vi "AI and AO.vi"(8 "error in (no error)":errorcluster, 10 "AO":waveform(dbl)[](array[waveform]), 11 "LockinDAQ in":refnum<class "LockinDAQ.lvclass">) -> (0 "error out":errorcluster, 2 "AI":waveform(dbl)[](array[waveform]), 3 "LockinDAQ out":refnum<class "LockinDAQ.lvclass">)   [LabVIEW 2016, in "LockinDAQ.lvclass"]
uses:
  LockinDAQ.lvclass
  LockinDAQ.lvclass/LockinDAQ.ctl
  <vilib>/DAQmx/read.llb/DAQmx Read (Analog 1D Wfm NChan NSamp).vi
  <vilib>/DAQmx/write.llb/DAQmx Write (Analog 1D Wfm NChan NSamp).vi
  <vilib>/DAQmx/miscellaneous.llb/DAQmx Fill In Error Info.vi
  <resource>/objmgr/daqmx.rc
panel:
  out "AvailSampPerChan 4":u32
  out "AvailSampPerChan 3":u32
  out "AvailSampPerChan 2":u32
  out "AvailSampPerChan 1":u32
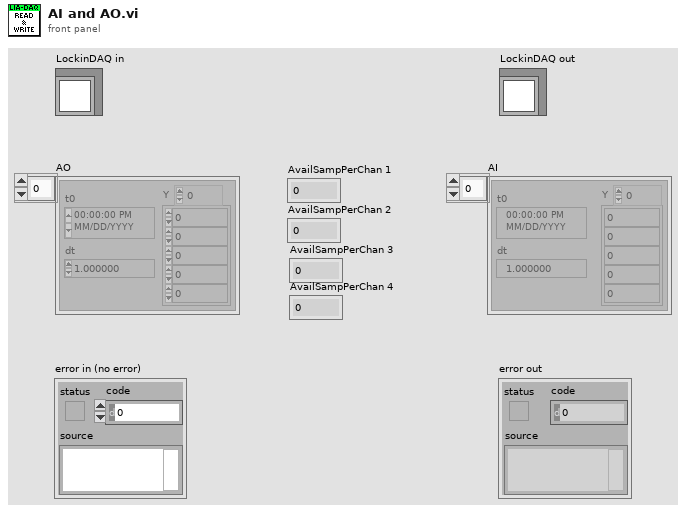
[diagram p1: front panel]
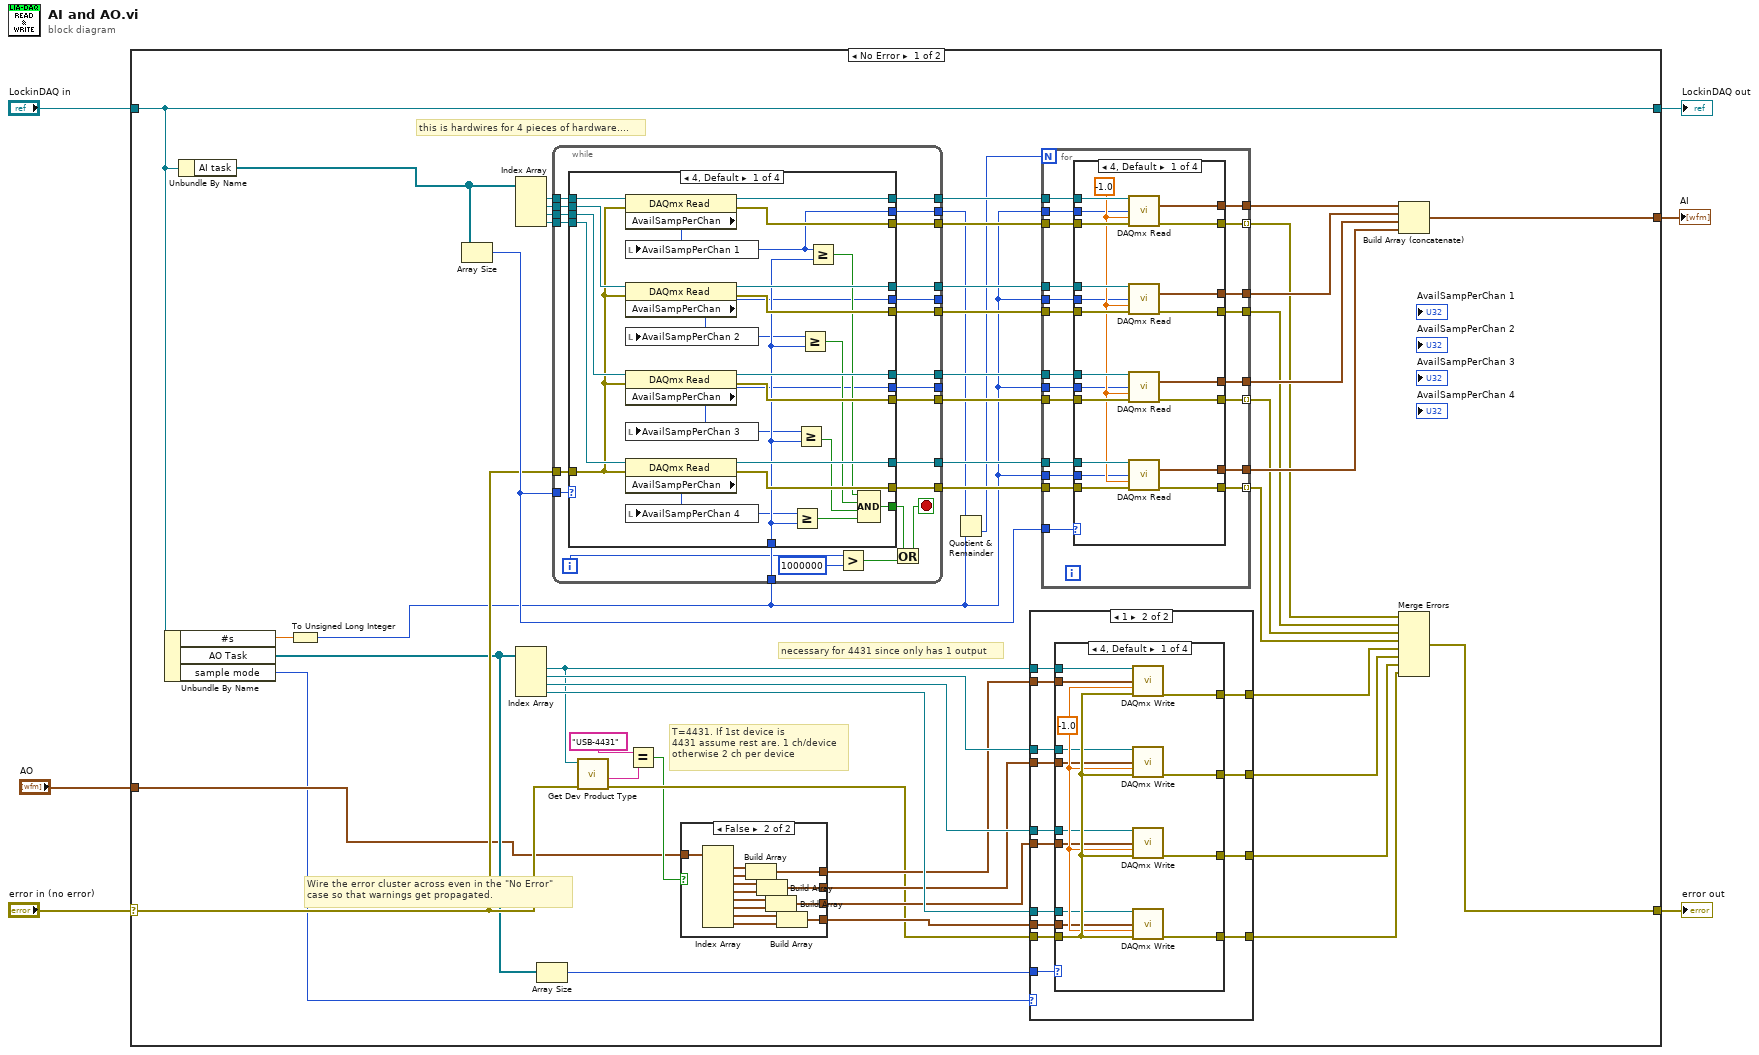
[diagram p0: block diagram]
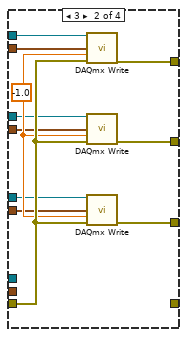
[diagram p3: hidden frame]
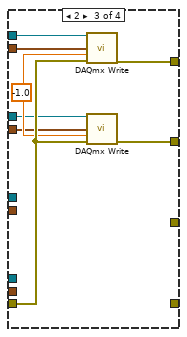
[diagram p4: hidden frame]
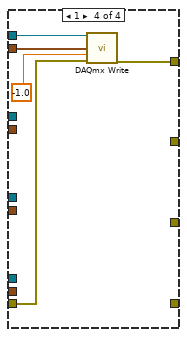
[diagram p5: hidden frame]
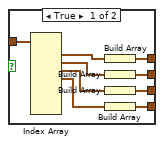
[diagram p6: hidden frame]
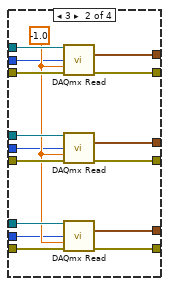
[diagram p7: hidden frame]
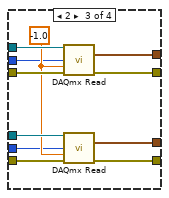
[diagram p8: hidden frame]
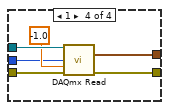
[diagram p9: hidden frame]
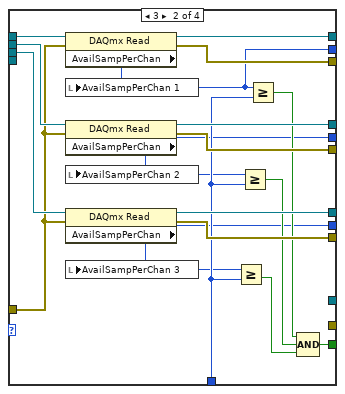
[diagram p10: hidden frame]
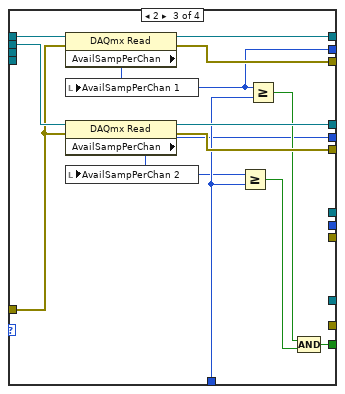
[diagram p11: hidden frame]
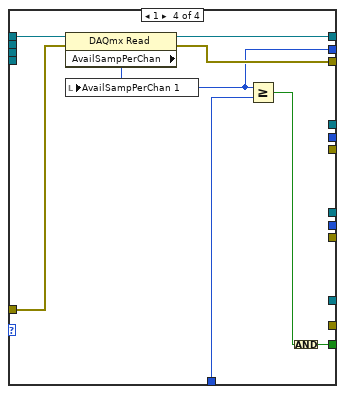
[diagram p12: hidden frame]
diagram:
  n1 = case shown="No Error" "error in (no error)" {
    selector: "error in (no error)" -> [w16 w292]
    tunnel: [w15 w292] -> w5
    tunnel: [w13 w291] -> w3
    tunnel: "LockinDAQ in" -> [w13 w291]
    tunnel: "AO" -> [w11 _]
    tunnel: [w10 _] -> w1
    frame No Error {
      # "this is hardwires for 4 pieces of hardware...."
      # "T=4431. If 1st device is \n4431 assume rest are. 1 ch/device\notherwise 2 ch per device"
      # "necessary for 4431 since only has 1 output"
      # "Wire the error cluster across even in the \"No Error\"\ncase so that warnings get propagated."
      n2 = Unbundle By Name(w13) -> ("#s"=w9:dbl, "AO Task"=w12:refnum<k21>[], "sample mode"=w7:i32)
      n3 = Unbundle By Name(w13) -> ("AI task"=w14:refnum<k21>[])
      n4 = To Unsigned Long Integer(number=w9) -> (unsigned 32bit integer=w8:u32)
      n5 = Array Size(array=w14) -> (size(s)=w21:i32)
      n6 = Index Array(array=w14) -> (element #1=w53:refnum<k21>, element #2=w54:refnum<k21>, element #3=w55:refnum<k21>, element #4=w56:refnum<k21>)  [unwired: 4 in]
      n7 = Index Array(array=w12) -> (element #1=w30:refnum<k21>, element #2=w44:refnum<k21>, element #3=w43:refnum<k21>, element #4=w42:refnum<k21>)  [unwired: 4 in]
      n8 = Array Size(array=w12) -> (size(s)=w31:i32)
      n9 = while {
        tunnel: w56 -> [w228]
        tunnel: w55 -> [w227]
        tunnel: w54 -> [w226]
        tunnel: w53 -> [w225]
        tunnel: [w224] -> w52
        tunnel: [w223] -> w51
        tunnel: [w222] -> w50
        tunnel: [w221] -> w49
        tunnel: w16 -> [w216]
        tunnel: [w220] -> w48
        tunnel: [w219] -> w47
        tunnel: [w218] -> w46
        tunnel: [w217] -> w45
        tunnel: w8 -> [w215]
        tunnel: [w212] -> w32
        tunnel: [w214] -> _
        tunnel: [w213] -> _
        tunnel: w21 -> [w211]
        i -> [w208]
        stop <- w209 stop-if-true
        n10 = case shown="4, Default" w211 {
          tunnel: w228 -> [w251 _ _ _]
          tunnel: w227 -> [w250 w269 _ _]
          tunnel: w226 -> [w249 w268 w282 _]
          tunnel: w225 -> [w248 w267 w281 w290]
          tunnel: [w247 w266 w280 w289] -> w224
          tunnel: [w246 w265 w279 _] -> w223
          tunnel: [w245 w264 _ _] -> w222
          tunnel: [w244 _ _ _] -> w221
          tunnel: [w243 w263 w278 w288] -> w220
          tunnel: [w242 w262 w277 _] -> w219
          tunnel: [w241 w261 _ _] -> w218
          tunnel: [w240 _ _ _] -> w217
          tunnel: w216 -> [w239 w260 w276 w287]
          tunnel: w215 -> [w234 w256 w273 w285]
          tunnel: [w229 w252 w270 w283] -> w210
          tunnel: [w232 w255 _ _] -> w214
          tunnel: [w231 w254 w272 _] -> w213
          tunnel: [w230 w253 w271 w284] -> w212
          frame 4, Default {
            n11 = property class="DAQmx Read"(reference=w248, error in=w239) -> (reference out=w247:refnum<k21>, error out=w243:errorcluster, "AvailSampPerChan"=w230:u32)
            n12 = local write "AvailSampPerChan 1"(w230) -> ()
            n13 = property class="DAQmx Read"(reference=w249, error in=w239) -> (reference out=w246:refnum<k21>, error out=w242:errorcluster, "AvailSampPerChan"=w231:u32)
            n14 = local write "AvailSampPerChan 2"(w231) -> ()
            n15 = property class="DAQmx Read"(reference=w250, error in=w239) -> (reference out=w245:refnum<k21>, error out=w241:errorcluster, "AvailSampPerChan"=w232:u32)
            n16 = local write "AvailSampPerChan 3"(w232) -> ()
            n17 = property class="DAQmx Read"(reference=w251, error in=w239) -> (reference out=w244:refnum<k21>, error out=w240:errorcluster, "AvailSampPerChan"=w233:u32)
            n18 = local write "AvailSampPerChan 4"(w233) -> ()
            n19 = Greater Or Equal?(x=w233, y=w234) -> (x >= y?=w238:bool)
            n20 = Greater Or Equal?(x=w232, y=w234) -> (x >= y?=w237:bool)
            n21 = Greater Or Equal?(x=w231, y=w234) -> (x >= y?=w236:bool)
            n22 = Greater Or Equal?(x=w230, y=w234) -> (x >= y?=w235:bool)
            n23 = Compound Arithmetic op=AND(w235, w236, w237, w238) -> (w229:bool)
          }
          frame 3 {
            n24 = property class="DAQmx Read"(reference=w267, error in=w260) -> (reference out=w266:refnum<k21>, error out=w263:errorcluster, "AvailSampPerChan"=w253:u32)
            n25 = local write "AvailSampPerChan 1"(w253) -> ()
            n26 = property class="DAQmx Read"(reference=w268, error in=w260) -> (reference out=w265:refnum<k21>, error out=w262:errorcluster, "AvailSampPerChan"=w254:u32)
            n27 = local write "AvailSampPerChan 2"(w254) -> ()
            n28 = property class="DAQmx Read"(reference=w269, error in=w260) -> (reference out=w264:refnum<k21>, error out=w261:errorcluster, "AvailSampPerChan"=w255:u32)
            n29 = local write "AvailSampPerChan 3"(w255) -> ()
            n30 = Greater Or Equal?(x=w255, y=w256) -> (x >= y?=w259:bool)
            n31 = Greater Or Equal?(x=w254, y=w256) -> (x >= y?=w258:bool)
            n32 = Greater Or Equal?(x=w253, y=w256) -> (x >= y?=w257:bool)
            n33 = Compound Arithmetic op=AND(w257, w258, w259) -> (w252:bool)
          }
          frame 2 {
            n34 = property class="DAQmx Read"(reference=w281, error in=w276) -> (reference out=w280:refnum<k21>, error out=w278:errorcluster, "AvailSampPerChan"=w271:u32)
            n35 = local write "AvailSampPerChan 1"(w271) -> ()
            n36 = property class="DAQmx Read"(reference=w282, error in=w276) -> (reference out=w279:refnum<k21>, error out=w277:errorcluster, "AvailSampPerChan"=w272:u32)
            n37 = local write "AvailSampPerChan 2"(w272) -> ()
            n38 = Greater Or Equal?(x=w272, y=w273) -> (x >= y?=w275:bool)
            n39 = Greater Or Equal?(x=w271, y=w273) -> (x >= y?=w274:bool)
            n40 = Compound Arithmetic op=AND(w274, w275) -> (w270:bool)
          }
          frame 1 {
            n41 = property class="DAQmx Read"(reference=w290, error in=w287) -> (reference out=w289:refnum<k21>, error out=w288:errorcluster, "AvailSampPerChan"=w284:u32)
            n42 = local write "AvailSampPerChan 1"(w284) -> ()
            n43 = Greater Or Equal?(x=w284, y=w285) -> (x >= y?=w286:bool)
            n44 = Compound Arithmetic op=AND(w286) -> (w283:bool)
          }
        }
        n45 = Greater?(x=w208, y=1000000) -> (0:w206:bool)
        n46 = Or(x=w210, y=w206) -> (x .or. y?=w209:bool)
      }
      n47 = call "Get Dev Product Type.vi"("error in (no error)"=w16, "Refnum in"=w30) -> ("error out"=w23:errorcluster, "ProductType"=w24:string)  [unwired: 6 in, 2 out]
      n48 = Equal?(x="USB-4431" ("ProductType"), y=w24) -> (x = y?=w22:bool)
      n49 = case shown="False" w22 {
        tunnel: [w117 w123] -> w27
        tunnel: [w116 w122] -> w28
        tunnel: [w115 w121] -> w29
        tunnel: [w113 w119] -> w26
        tunnel: w11 -> [w112 w118]
        frame True {
          n50 = Index Array(array=w112) -> (element #1=w114:waveform(dbl), element #2=w111:waveform(dbl), element #3=w110:waveform(dbl), element #4=w109:waveform(dbl))  [unwired: 8 in, 4 out]
          n51 = Build Array(w114) -> (w113:waveform(dbl)[])
          n52 = Build Array(w111) -> (w117:waveform(dbl)[])
          n53 = Build Array(w110) -> (w116:waveform(dbl)[])
          n54 = Build Array(w109) -> (w115:waveform(dbl)[])
        }
        frame False {
          n55 = Index Array(array=w118) -> (element #1=w120:waveform(dbl), element #2=w130:waveform(dbl), element #3=w129:waveform(dbl), element #4=w128:waveform(dbl), element #5=w127:waveform(dbl), element #6=w126:waveform(dbl), element #7=w125:waveform(dbl), element #8=w124:waveform(dbl))  [unwired: 8 in]
          n56 = Build Array(w120, w130) -> (w119:waveform(dbl)[])
          n57 = Build Array(w129, w128) -> (w123:waveform(dbl)[])
          n58 = Build Array(w127, w126) -> (w122:waveform(dbl)[])
          n59 = Build Array(w125, w124) -> (w121:waveform(dbl)[])
        }
      }
      n60 = Quotient & Remainder(x=w32, y=w8) -> (floor(x/y)=w33:u32)  [unwired: 1 out]
      n61 = case shown="1" w7 {
        tunnel: w44 -> [_ w70]
        tunnel: w43 -> [_ w69]
        tunnel: w42 -> [_ w68]
        tunnel: [_ w67] -> w41
        tunnel: [_ w66] -> w40
        tunnel: [_ w65] -> w39
        tunnel: [_ w64] -> w38
        tunnel: w31 -> [_ w63]
        tunnel: w30 -> [_ w62]
        tunnel: w29 -> [_ w61]
        tunnel: w28 -> [_ w60]
        tunnel: w27 -> [_ w59]
        tunnel: w26 -> [_ w58]
        tunnel: w23 -> [_ w57]
        frame 0, Default {
          # "0 = finite sample mode (IV\nmode). Do not try to write\nmore samples to the buffer"
        }
        frame 1 {
          n62 = case shown="4, Default" w63 {
            tunnel: w57 -> [w84 w95 w103 w108]
            tunnel: w70 -> [w82 w93 w101 _]
            tunnel: w69 -> [w81 w92 _ _]
            tunnel: w68 -> [w80 _ _ _]
            tunnel: w59 -> [w79 w91 w100 _]
            tunnel: w60 -> [w78 w90 _ _]
            tunnel: w61 -> [w77 _ _ _]
            tunnel: [w76 w89 w99 w106] -> w67
            tunnel: [w75 w88 w98 _] -> w66
            tunnel: [w74 w87 _ _] -> w65
            tunnel: [w73 _ _ _] -> w64
            tunnel: w62 -> [w72 w86 w97 w105]
            tunnel: w58 -> [w71 w85 w96 w104]
            frame 4, Default {
              w83 = -1.0 ("timeout")
              n63 = call-poly <vilib>:"DAQmx Write.vi"("task/channels in"=w72, "data"=w71, "timeout"=w83, "error in"=w84) -> ("error out"=w76:errorcluster)  [unwired: 9 in, 2 out]
              n64 = call-poly <vilib>:"DAQmx Write.vi"("task/channels in"=w82, "data"=w79, "timeout"=w83, "error in"=w84) -> ("error out"=w75:errorcluster)  [unwired: 9 in, 2 out]
              n65 = call-poly <vilib>:"DAQmx Write.vi"("task/channels in"=w81, "data"=w78, "timeout"=w83, "error in"=w84) -> ("error out"=w74:errorcluster)  [unwired: 9 in, 2 out]
              n66 = call-poly <vilib>:"DAQmx Write.vi"("task/channels in"=w80, "data"=w77, "timeout"=w83, "error in"=w84) -> ("error out"=w73:errorcluster)  [unwired: 9 in, 2 out]
            }
            frame 3 {
              w94 = -1.0 ("timeout")
              n67 = call-poly <vilib>:"DAQmx Write.vi"("task/channels in"=w86, "data"=w85, "timeout"=w94, "error in"=w95) -> ("error out"=w89:errorcluster)  [unwired: 9 in, 2 out]
              n68 = call-poly <vilib>:"DAQmx Write.vi"("task/channels in"=w93, "data"=w91, "timeout"=w94, "error in"=w95) -> ("error out"=w88:errorcluster)  [unwired: 9 in, 2 out]
              n69 = call-poly <vilib>:"DAQmx Write.vi"("task/channels in"=w92, "data"=w90, "timeout"=w94, "error in"=w95) -> ("error out"=w87:errorcluster)  [unwired: 9 in, 2 out]
            }
            frame 2 {
              w102 = -1.0 ("timeout")
              n70 = call-poly <vilib>:"DAQmx Write.vi"("task/channels in"=w97, "data"=w96, "timeout"=w102, "error in"=w103) -> ("error out"=w99:errorcluster)  [unwired: 9 in, 2 out]
              n71 = call-poly <vilib>:"DAQmx Write.vi"("task/channels in"=w101, "data"=w100, "timeout"=w102, "error in"=w103) -> ("error out"=w98:errorcluster)  [unwired: 9 in, 2 out]
            }
            frame 1 {
              n72 = call-poly <vilib>:"DAQmx Write.vi"("task/channels in"=w105, "data"=w104, "timeout"=-1.0, "error in"=w108) -> ("error out"=w106:errorcluster)  [unwired: 9 in, 2 out]
            }
          }
        }
      }
      n73 = for {
        N: w33 -> [_]
        tunnel: w52 -> [w151]
        tunnel: w51 -> [w150]
        tunnel: w50 -> [w149]
        tunnel: w49 -> [w148]
        tunnel: w48 -> [w147]
        tunnel: w47 -> [w146]
        tunnel: w46 -> [w145]
        tunnel: w45 -> [w144]
        tunnel: [w143] -> w37
        tunnel: [w142] -> w36
        tunnel: [w141] -> w35
        tunnel: [w140] -> w34
        tunnel: w8 -> [w139]
        tunnel: w8 -> [w138]
        tunnel: w8 -> [w137]
        tunnel: w8 -> [w136]
        tunnel: [w135] -> w18 mode=indexing
        tunnel: [w134] -> w19
        tunnel: [w133] -> w20 mode=indexing
        tunnel: [w132] -> w17 mode=indexing
        tunnel: w21 -> [w131]
        n74 = case shown="4, Default" w131 {
          tunnel: w151 -> [w172 w188 w199 w205]
          tunnel: w150 -> [w171 w187 w198 _]
          tunnel: w149 -> [w170 w186 _ _]
          tunnel: w148 -> [w169 _ _ _]
          tunnel: w147 -> [w168 w185 w197 w204]
          tunnel: w146 -> [w167 w184 w196 _]
          tunnel: w145 -> [w166 w183 _ _]
          tunnel: w144 -> [w165 _ _ _]
          tunnel: [w163 w181 w194 _] -> w143
          tunnel: [w162 w180 w193 w202] -> w142
          tunnel: [w161 w179 _ _] -> w141
          tunnel: [w160 _ _ _] -> w140
          tunnel: w139 -> [w159 _ _ _]
          tunnel: w138 -> [w158 w178 w192 w201]
          tunnel: w137 -> [w157 w177 _ _]
          tunnel: w136 -> [w156 w176 w191 _]
          tunnel: [w155 w175 w190 w200] -> w135
          tunnel: [w154 w174 w189 _] -> w134
          tunnel: [w153 w173 _ _] -> w133
          tunnel: [w152 _ _ _] -> w132
          frame 4, Default {
            w164 = -1.0 ("timeout")
            n75 = call-poly <vilib>:"DAQmx Read.vi"("task/channels in"=w172, "number of samples per channel"=w158, "timeout"=w164, "error in"=w168) -> ("data"=w162:waveform(dbl)[], "error out"=w155:errorcluster)  [unwired: 9 in, 1 out]
            n76 = call-poly <vilib>:"DAQmx Read.vi"("task/channels in"=w171, "number of samples per channel"=w156, "timeout"=w164, "error in"=w167) -> ("data"=w163:waveform(dbl)[], "error out"=w154:errorcluster)  [unwired: 9 in, 1 out]
            n77 = call-poly <vilib>:"DAQmx Read.vi"("task/channels in"=w170, "number of samples per channel"=w157, "timeout"=w164, "error in"=w166) -> ("data"=w161:waveform(dbl)[], "error out"=w153:errorcluster)  [unwired: 9 in, 1 out]
            n78 = call-poly <vilib>:"DAQmx Read.vi"("task/channels in"=w169, "number of samples per channel"=w159, "timeout"=w164, "error in"=w165) -> ("data"=w160:waveform(dbl)[], "error out"=w152:errorcluster)  [unwired: 9 in, 1 out]
          }
          frame 3 {
            w182 = -1.0 ("timeout")
            n79 = call-poly <vilib>:"DAQmx Read.vi"("task/channels in"=w188, "number of samples per channel"=w178, "timeout"=w182, "error in"=w185) -> ("data"=w180:waveform(dbl)[], "error out"=w175:errorcluster)  [unwired: 9 in, 1 out]
            n80 = call-poly <vilib>:"DAQmx Read.vi"("task/channels in"=w187, "number of samples per channel"=w176, "timeout"=w182, "error in"=w184) -> ("data"=w181:waveform(dbl)[], "error out"=w174:errorcluster)  [unwired: 9 in, 1 out]
            n81 = call-poly <vilib>:"DAQmx Read.vi"("task/channels in"=w186, "number of samples per channel"=w177, "timeout"=w182, "error in"=w183) -> ("data"=w179:waveform(dbl)[], "error out"=w173:errorcluster)  [unwired: 9 in, 1 out]
          }
          frame 2 {
            w195 = -1.0 ("timeout")
            n82 = call-poly <vilib>:"DAQmx Read.vi"("task/channels in"=w199, "number of samples per channel"=w192, "timeout"=w195, "error in"=w197) -> ("data"=w193:waveform(dbl)[], "error out"=w190:errorcluster)  [unwired: 9 in, 1 out]
            n83 = call-poly <vilib>:"DAQmx Read.vi"("task/channels in"=w198, "number of samples per channel"=w191, "timeout"=w195, "error in"=w196) -> ("data"=w194:waveform(dbl)[], "error out"=w189:errorcluster)  [unwired: 9 in, 1 out]
          }
          frame 1 {
            n84 = call-poly <vilib>:"DAQmx Read.vi"("task/channels in"=w205, "number of samples per channel"=w201, "timeout"=-1.0, "error in"=w204) -> ("data"=w202:waveform(dbl)[], "error out"=w200:errorcluster)  [unwired: 9 in, 1 out]
          }
        }
      }
      n85 = Build Array (concatenate)(w36, w37, w35, w34) -> (w10:waveform(dbl)[])
      n86 = Merge Errors(w18, w19, w20, w17, w41, w40, w39, w38) -> (w15:errorcluster)
    }
    frame Error {
    }
  }
  "error out" <- w5
  "LockinDAQ out" <- w3
  "AI" <- w1
